vi "Generate Programmatic Build Command Line String.vi"() -> ()   [LabVIEW 2023]
doc: "This example shows how to use the Application:Command Line Arguments property to retrieve parameters that were returned when the LabVIEW executable was called from the command line. Those parameters are then passed to the Build.vi to programmatically build an executable based on a build specification in the specified project."
panel:
  out "Command Line String":string
  # "Overview: Demonstrates how to programmatically execute a build specification from the command line with the Application Builder VIs.\nRequirements: LabVIEW Professional Development System or LabVIEW Application Builder\nInstructions:\n1. Run the VI to generate a command line string that will programmatically execute a build specification.\n2. Highlight the text in the Command Line String indicator and select Edit > Copy to copy the text to the clipboard.\n3. Exit LabVIEW.\n4. Paste the string into a command line window and run the command. (To do this on Windows, press Window-R, type 'cmd', press Enter, right-click in the command window and select Paste, then press Enter.)"
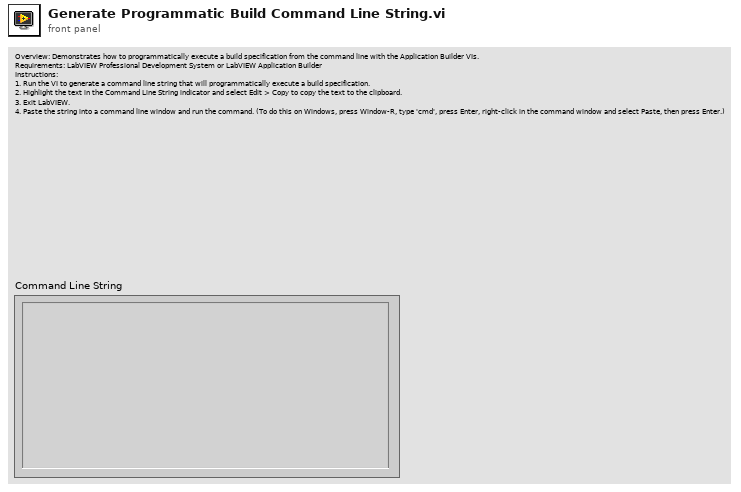
[diagram p1: front panel]
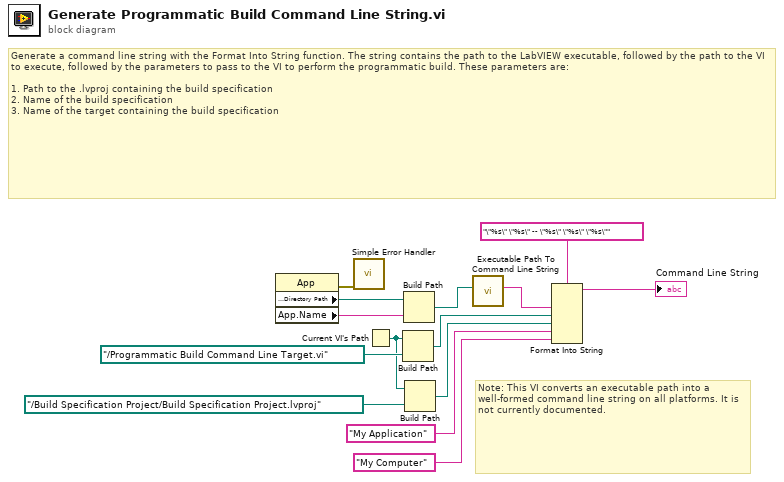
[diagram p0: block diagram]
diagram:
  # "Note: This VI converts an executable path into a well-formed command line string on all platforms. It is not currently documented."
  # "Generate a command line string with the Format Into String function. The string contains the path to the LabVIEW executable, followed by the path to the VI to execute, followed by the parameters to pass to the VI to perform the programmatic build. These parameters are:\n\n1. Path to the .lvproj containing the build specification\n2. Name of the build specification\n3. Name of the target containing the build specification"
  n1 = property class="App"() -> (error out=w13:errorcluster, "Application:Directory Path"=w12:path, "App.Name"=w11:string)  [unwired: 2 in, 1 out]
  n2 = call <vilib>:"Simple Error Handler.vi"("error in (no error)"=w13) -> ()  [unwired: 1 in, 8 out]
  n3 = Current VI's Path() -> (path=w7:path)
  n4 = Build Path(base path=w7, name or relative path=path "../Programmatic Build Command Line Target.vi" ("path")) -> (appended path=w9:path)
  n5 = Build Path(base path=w12, name or relative path=w11) -> (appended path=w2:path)
  n6 = Build Path(base path=w7, name or relative path=path "../Build Specification Project/Build Specification Project.lvproj" ("path")) -> (appended path=w5:path)
  n7 = call <vilib>:"Executable Path To Command Line String.vi"("Executable Path"=w2) -> ("System Exec String"=w1:string)  [unwired: 10 in]
  n8 = Format Into String(format string="\"%s\" \"%s\" -- \"%s\" \"%s\" \"%s\"", w1, w9, w5, "My Application", "My Computer") -> (resulting string=→"Command Line String":string)  [unwired: 2 in, 1 out]
